vi "asset.create_add_label.vi"(8 "error in":errorcluster, 11 "AssetCreateStaging in":refnum<class "AssetCreateStaging.lvclass">) -> (0 "error out":errorcluster, 3 "AssetCreateStaging out":refnum<class "AssetCreateStaging.lvclass">)   [LabVIEW 2020, in "AssetCreateStaging.lvclass"]
doc: "Adds a label to the asset being created."
uses:
  AssetCreateStaging.lvclass
  AssetCreateStaging.lvclass/AssetCreateStaging.ctl
  client.lvlib
panel:
  in  "label":string
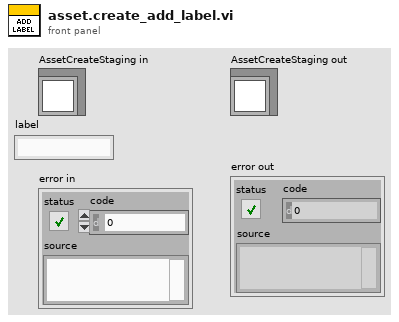
[diagram p1: front panel]
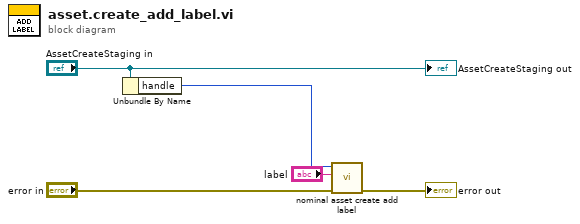
[diagram p0: block diagram]
diagram:
  n1 = Unbundle By Name("AssetCreateStaging in") -> ("handle"=w3:i32)
  n2 = call "nominal asset create add label.vi"("error in (no error)"="error in", "label"="label", "staging"=w3) -> ("error out"=→"error out":errorcluster)  [unwired: 7 in, 1 out]
  "AssetCreateStaging out" <- "AssetCreateStaging in"
